vi "tb_fft test_host_sgl_2points.vi"() -> ()   [LabVIEW 2011]
uses:
  <userlib>/FPGA Library/Code Development/Signal Processing/FFT Block/FFT/Controls/FFT States.ctl
  <userlib>/FPGA Library/Code Development/Signal Processing/FFT Block/FFT/FFT Size.ctl
  <vilib>/Analysis/2dsp.llb/Real FFT.vi
  <vilib>/measure/maspectr.llb/FFT Spectrum (Mag-Phase) for 1 Chan (CDB).vi
  <vilib>/Analysis/1siggen.llb/Ramp Pattern by Samples.vi
  <vilib>/Analysis/NI_AALBase.lvlib
  <vilib>/measure/NI_MAPro.lvlib
  <vilib>/Analysis/NI_AALPro.lvlib
panel:
  out "xk_index":fxp<+,9,9>
  out "FFT Output Index":i32
  out "Current Index":u16
  out "Current State":T1=enum."Process"
  out "LabVIEW FPGA OUt":dbl[](array[numeric])
  out "LabVIEW":dbl[](array[numeric])
  out "Output":dbl[](array[numeric])
  out "Iterations Done":i32=550
  out "Pass?":bool=TRUE
  out "Error Signal":dbl[](graph)=[-2.3209475248815725e-14, 2.842170943040401e-14, -1.423246383868342e-14, -5.0290155712318274e-15, -5.617693635462835e-15, -1.2654220787659285e-14, -2.2653800450034258e-15, -7.817855587735912e-15, -5.642048551852787e-16, -4.848122315266641e-15, -1.4066308379314257e-15, -5.26182206995493e-15, -1.6787700245303399e-15, -3.5317597533564052e-15, -1.2179408859273234e-15, -5.682239243846926e-16, -1.476012201472354e-15, -4.387189911370367e-15, -4.712784380658982e-16, -1.1279118711067195e-15, -8.457455385367502e-16, -1.7591217350674133e-15, -1.2234105719754893e-15, -3.1796619632735843e-15, -1.1311752817825782e-15, -7.652138728201138e-16, -4.95475236507169e-16, -1.3804968391458857e-15, -6.200872213680143e-16, -1.6208905183375611e-15, -7.900785734892874e-16, -6.215416191232572e-15, -3.6014963741383564e-16, -6.5735506151035904e-15, -5.438526124809484e-16, -8.859964049951827e-16, -4.660820542011352e-16, -4.331250169872678e-16, -5.070423607357574e-16, -1.334222221931296e-15, -4.161038840225869e-16, -2.162642520615897e-15, -4.832602196126579e-16, -1.8466113911920694e-15, -5.111720910128212e-16, -1.3077661139157257e-15, -1.317295841380055e-16, -1.5344645445695557e-15, -5.003143032383381e-16, -8.907780307170318e-16, -3.4910614331552773e-16, -1.9659375815054982e-15, -2.522820868197333e-16, -1.3494997210405505e-15, -2.1367142635572254e-16, -1.2649677550390071e-15, -3.5078397942125153e-16, -1.493960591155926e-15, -3.7008746035102686e-16, -2.5695474807823932e-15, -2.1842124513731103e-16, -1.682876439042557e-15, -4.96013146890552e-16, -6.5726931140504286e-15, -2.3111578430367925e-16, -5.778724315304478e-15, -1.7672272640256473e-16, -2.3917285436809857e-15, -8.413654196767352e-17, -2.1045096122203425e-15, -2.324245509223888e-16, -2.1899677460894678e-15, -2.7245802781795665e-16, -1.0471757725153366e-15, -2.6086976997519237e-16, -2.7751674747999853e-15, -3.5068777984061774e-16, -1.4999120779771695e-15, -5.776639758822378e-17, -1.865769852058881e-15, -3.141749171548091e-16, -1.442932533559895e-15, -3.715679972475205e-16, -2.4873545340143905e-15, -3.0316037042699785e-16, -1.37060843732013e-15, -3.432134673273237e-17, -2.1823140172583753e-15, -3.2893911942517435e-16, -1.3802374497384821e-15, -2.515468723190618e-16, -2.0407080560795774e-15, -7.825246283752062e-17, -9.605012681453347e-16, -1.6665822022539347e-16, -8.585854605590916e-15, -8.279239838517457e-17, -8.029942062406046e-15, -2.549866803230553e-16, -1.3304883103107788e-15, -2.90011130209677e-16, -2.5843153744562437e-16, -3.0946190583309643e-16, -1.5925989429078613e-15, -1.9088697868535118e-16, -1.0709404142245489e-15, -1.863213961293967e-16, -1.401179966237845e-15, -4.025510697204942e-16, -3.065000004186774e-16, -2.4056748095016175e-16, -3.564162060583895e-15, -9.550773452918578e-17, -3.8814679519282134e-15, -6.671123007721539e-17, -5.082068342041713e-16, -1.8944012535004732e-16, -1.0775874498436763e-15, -2.0329123879890962e-16, -2.241124999344413e-15, -1.8315131472796022e-16, -2.5293144435025902e-15, -2.3090799989339955e-16, -2.612178765857882e-15, -7.52239796616572e-17, -1.3979455926566411e-15, -2.5913851848827294e-16, -7.112961996896967e-15, -2.225733614385263e-16, -7.158697954722229e-15, -2.1660085057067423e-16, -2.6486921612808084e-15, -6.056613111055876e-17, -2.288188675935301e-15, -2.574708219682569e-16, -9.746365606310544e-16, -2.5811420637914955e-16, -8.308310394594462e-16, -4.494030496521331e-17, -1.4914047073883096e-15, -1.2275946211757026e-16, -2.6789082049114747e-15, -7.646153710119143e-17, -3.614594974384435e-15, -1.5957370718388087e-16, -2.9071637037790352e-15, -1.0273012860538455e-16, -1.3529679760932233e-15, -2.1337438724207498e-16, -2.366087417632634e-15, -9.550540044778412e-17, -1.5267377900302278e-15, -1.0388147266081965e-16, -2.509352775164673e-15, -2.3294021415221696e-16, -1.5871319492314687e-15, -1.629641167659651e-16, -3.155068388354255e-15, -2.4295533381250624e-16, -1.789790942017654e-15, -2.1957682081227828e-16, -2.0620909489757014e-15, -2.636517897912316e-16, -3.19876498904266e-15, -4.76024074878868e-17, -2.8623217823864246e-15, -2.340225419378271e-16, -2.720367262450368e-15, -2.798717011154696e-16, -3.2704501244531444e-15, -8.294783416780197e-17, -4.3774499283332104e-15, -6.583259151313607e-17, -1.9123572024036315e-15, -8.859554359303103e-17, -3.909561650717318e-15, -2.157753926548324e-16, -2.631616832513605e-15, -1.8282424749852087e-16, -1.5012598370928595e-15, -2.6297488382582883e-16, -2.739819934401838e-16, -2.1835568909079528e-16, -4.566965697604556e-16, -2.844726135635231e-16, -6.029898128165984e-16, -4.031968136940985e-16, -1.2254274776086847e-15, -1.8567128477488958e-16, -1.2812099893063057e-15, -9.450275719635022e-17, -5.96208200198294e-15, -1.7413014862493185e-16, -6.362837003873818e-15, -3.8442560991005193e-16, -8.511897473684678e-16, -3.0298323627896944e-16, -6.374617717285576e-16, -3.980117316625464e-17, -1.889994438645939e-15, -7.924595323298657e-17, -1.1680802186811143e-15, -1.513694447821511e-16, -3.626366865071199e-16, -4.1911022380985105e-16, -1.5491215798532264e-15, -3.3152634782517783e-16, -1.0511118915755967e-15, -2.8375241753187317e-16, -3.0041210935611057e-15, -2.312884286263144e-16, -8.680462300544733e-16, -5.913378666039998e-16, -2.0124813913536014e-15, -4.849627295200987e-16, -3.0245786651048457e-15, -2.562926943075326e-16, -9.586214531000217e-16, -7.630416896386312e-17, -1.885296996390658e-15, -3.7641062798780547e-16, -1.3322161170514853e-15, -6.258042048959739e-16, -2.9484061140259706e-15, -2.478244140346566e-16, -4.381349750736086e-15, -3.055345357451583e-16, -8.254308413688034e-16, -2.1611396728793227e-16, -2.100174130362261e-15, -5.639679223541525e-16, -2.039042989477575e-15, -7.356320721078596e-16, -2.155129637976514e-15, -2.917622859196026e-16, -2.9817337018338868e-15, -5.901631083403165e-17, -1.4257302964464585e-15, -5.707161677436202e-16, -1.3123195162261534e-15, -1.3214037338257707e-15, -3.0060428009987197e-15, -9.650139214557572e-16, -2.010017297160963e-15, -9.477531974798123e-16, -4.598043857065251e-15, -1.2635405532302e-15, -5.575592142985788e-15, -1.2288406491237445e-15, -2.1260965321182736e-15, -1.1476659587055287e-15, -1.4004468922647886e-14, -1.8926642492776802e-15, -5.2356515256904374e-15, -7.733954207320486e-15, -3.0001115817680726e-14, -2.8911741707313143e-15, -3.0001115817680726e-14, -7.733954207320486e-15, -5.2356515256904374e-15, -1.8926642492776802e-15, -1.4004468922647886e-14, -1.1476659587055287e-15, -2.1260965321182736e-15, -1.2288406491237445e-15, -5.575592142985788e-15, -1.2635405532302e-15, -4.598043857065251e-15, -9.477531974798123e-16, -2.010017297160963e-15, -9.650139214557572e-16, -3.0060428009987197e-15, -1.3214037338257707e-15, -1.3123195162261534e-15, -5.707161677436202e-16, -1.4257302964464585e-15, -5.901631083403165e-17, -2.9817337018338868e-15, -2.917622859196026e-16, -2.155129637976514e-15, -7.356320721078596e-16, -2.039042989477575e-15, -5.639679223541525e-16, -2.100174130362261e-15, -2.1611396728793227e-16, -8.254308413688034e-16, -3.055345357451583e-16, -4.381349750736086e-15, -2.478244140346566e-16, -2.9484061140259706e-15, -6.258042048959739e-16, -1.3322161170514853e-15, -3.7641062798780547e-16, -1.885296996390658e-15, -7.630416896386312e-17, -9.586214531000217e-16, -2.562926943075326e-16, -3.0245786651048457e-15, -4.849627295200987e-16, -2.0124813913536014e-15, -5.913378666039998e-16, -8.680462300544733e-16, -2.312884286263144e-16, -3.0041210935611057e-15, -2.8375241753187317e-16, -1.0511118915755967e-15, -3.3152634782517783e-16, -1.5491215798532264e-15, -4.1911022380985105e-16, -3.626366865071199e-16, -1.513694447821511e-16, -1.1680802186811143e-15, -7.924595323298657e-17, -1.889994438645939e-15, -3.980117316625464e-17, -6.374617717285576e-16, -3.0298323627896944e-16, -8.511897473684678e-16, -3.8442560991005193e-16, -6.362837003873818e-15, -1.7413014862493185e-16, -5.96208200198294e-15, -9.450275719635022e-17, -1.2812099893063057e-15, -1.8567128477488958e-16, -1.2254274776086847e-15, -4.031968136940985e-16, -6.029898128165984e-16, -2.844726135635231e-16, -4.566965697604556e-16, -2.1835568909079528e-16, -2.739819934401838e-16, -2.6297488382582883e-16, -1.5012598370928595e-15, -1.8282424749852087e-16, -2.631616832513605e-15, -2.157753926548324e-16, -3.909561650717318e-15, -8.859554359303103e-17, -1.9123572024036315e-15, -6.583259151313607e-17, -4.3774499283332104e-15, -8.294783416780197e-17, -3.2704501244531444e-15, -2.798717011154696e-16, -2.720367262450368e-15, -2.340225419378271e-16, -2.8623217823864246e-15, -4.76024074878868e-17, -3.19876498904266e-15, -2.636517897912316e-16, -2.0620909489757014e-15, -2.1957682081227828e-16, -1.789790942017654e-15, -2.4295533381250624e-16, -3.155068388354255e-15, -1.629641167659651e-16, -1.5871319492314687e-15, -2.3294021415221696e-16, -2.509352775164673e-15, -1.0388147266081965e-16, -1.5267377900302278e-15, -9.550540044778412e-17, -2.366087417632634e-15, -2.1337438724207498e-16, -1.3529679760932233e-15, -1.0273012860538455e-16, -2.9071637037790352e-15, -1.5957370718388087e-16, -3.614594974384435e-15, -7.646153710119143e-17, -2.6789082049114747e-15, -1.2275946211757026e-16, -1.4914047073883096e-15, -4.494030496521331e-17, -8.308310394594462e-16, -2.5811420637914955e-16, -9.746365606310544e-16, -2.574708219682569e-16, -2.288188675935301e-15, -6.056613111055876e-17, -2.6486921612808084e-15, -2.1660085057067423e-16, -7.158697954722229e-15, -2.225733614385263e-16, -7.112961996896967e-15, -2.5913851848827294e-16, -1.3979455926566411e-15, -7.52239796616572e-17, -2.612178765857882e-15, -2.3090799989339955e-16, -2.5293144435025902e-15, -1.8315131472796022e-16, -2.241124999344413e-15, -2.0329123879890962e-16, -1.0775874498436763e-15, -1.8944012535004732e-16, -5.082068342041713e-16, -6.671123007721539e-17, -3.8814679519282134e-15, -9.550773452918578e-17, -3.564162060583895e-15, -2.4056748095016175e-16, -3.065000004186774e-16, -4.025510697204942e-16, -1.401179966237845e-15, -1.863213961293967e-16, -1.0709404142245489e-15, -1.9088697868535118e-16, -1.5925989429078613e-15, -3.0946190583309643e-16, -2.5843153744562437e-16, -2.90011130209677e-16, -1.3304883103107788e-15, -2.549866803230553e-16, -8.029942062406046e-15, -8.279239838517457e-17, -8.585854605590916e-15, -1.6665822022539347e-16, -9.605012681453347e-16, -7.825246283752062e-17, -2.0407080560795774e-15, -2.515468723190618e-16, -1.3802374497384821e-15, -3.2893911942517435e-16, -2.1823140172583753e-15, -3.432134673273237e-17, -1.37060843732013e-15, -3.0316037042699785e-16, -2.4873545340143905e-15, -3.715679972475205e-16, -1.442932533559895e-15, -3.141749171548091e-16, -1.865769852058881e-15, -5.776639758822378e-17, -1.4999120779771695e-15, -3.5068777984061774e-16, -2.7751674747999853e-15, -2.6086976997519237e-16, -1.0471757725153366e-15, -2.7245802781795665e-16, -2.1899677460894678e-15, -2.324245509223888e-16, -2.1045096122203425e-15, -8.413654196767352e-17, -2.3917285436809857e-15, -1.7672272640256473e-16, -5.778724315304478e-15, -2.3111578430367925e-16, -6.5726931140504286e-15, -4.96013146890552e-16, -1.682876439042557e-15, -2.1842124513731103e-16, -2.5695474807823932e-15, -3.7008746035102686e-16, -1.493960591155926e-15, -3.5078397942125153e-16, -1.2649677550390071e-15, -2.1367142635572254e-16, -1.3494997210405505e-15, -2.522820868197333e-16, -1.9659375815054982e-15, -3.4910614331552773e-16, -8.907780307170318e-16, -5.003143032383381e-16, -1.5344645445695557e-15, -1.317295841380055e-16, -1.3077661139157257e-15, -5.111720910128212e-16, -1.8466113911920694e-15, -4.832602196126579e-16, -2.162642520615897e-15, -4.161038840225869e-16, -1.334222221931296e-15, -5.070423607357574e-16, -4.331250169872678e-16, -4.660820542011352e-16, -8.859964049951827e-16, -5.438526124809484e-16, -6.5735506151035904e-15, -3.6014963741383564e-16, -6.215416191232572e-15, -7.900785734892874e-16, -1.6208905183375611e-15, -6.200872213680143e-16, -1.3804968391458857e-15, -4.95475236507169e-16, -7.652138728201138e-16, -1.1311752817825782e-15, -3.1796619632735843e-15, -1.2234105719754893e-15, -1.7591217350674133e-15, -8.457455385367502e-16, -1.1279118711067195e-15, -4.712784380658982e-16, -4.387189911370367e-15, -1.476012201472354e-15, -5.682239243846926e-16, -1.2179408859273234e-15, -3.5317597533564052e-15, -1.6787700245303399e-15, -5.26182206995493e-15, -1.4066308379314257e-15, -4.848122315266641e-15, -5.642048551852787e-16, -7.817855587735912e-15, -2.2653800450034258e-15, -1.2654220787659285e-14, -5.617693635462835e-15, -5.0290155712318274e-15, -1.423246383868342e-14, 2.842170943040401e-14]
  out "FFT_FLP_LabVIEW":dbl[](graph)
  out "LabVIEW FPGA":dbl[](graph)=[0.0, 256.0, 0.0, 0.0, 0.0, 0.0, 0.0, 0.0, 0.0, 0.0, 0.0, 0.0, 0.0, 0.0, 0.0, 0.0, 0.0, 0.0, 0.0, 0.0, 0.0, 0.0, 0.0, 0.0, 0.0, 0.0, 0.0, 0.0, 0.0, 0.0, 0.0, 0.0, 0.0, 0.0, 0.0, 0.0, 0.0, 0.0, 0.0, 0.0, 0.0, 0.0, 0.0, 0.0, 0.0, 0.0, 0.0, 0.0, 0.0, 0.0, 0.0, 0.0, 0.0, 0.0, 0.0, 0.0, 0.0, 0.0, 0.0, 0.0, 0.0, 0.0, 0.0, 0.0, 0.0, 0.0, 0.0, 0.0, 0.0, 0.0, 0.0, 0.0, 0.0, 0.0, 0.0, 0.0, 0.0, 0.0, 0.0, 0.0, 0.0, 0.0, 0.0, 0.0, 0.0, 0.0, 0.0, 0.0, 0.0, 0.0, 0.0, 0.0, 0.0, 0.0, 0.0, 0.0, 0.0, 0.0, 0.0, 0.0, 0.0, 0.0, 0.0, 0.0, 0.0, 0.0, 0.0, 0.0, 0.0, 0.0, 0.0, 0.0, 0.0, 0.0, 0.0, 0.0, 0.0, 0.0, 0.0, 0.0, 0.0, 0.0, 0.0, 0.0, 0.0, 0.0, 0.0, 0.0, 0.0, 0.0, 0.0, 0.0, 0.0, 0.0, 0.0, 0.0, 0.0, 0.0, 0.0, 0.0, 0.0, 0.0, 0.0, 0.0, 0.0, 0.0, 0.0, 0.0, 0.0, 0.0, 0.0, 0.0, 0.0, 0.0, 0.0, 0.0, 0.0, 0.0, 0.0, 0.0, 0.0, 0.0, 0.0, 0.0, 0.0, 0.0, 0.0, 0.0, 0.0, 0.0, 0.0, 0.0, 0.0, 0.0, 0.0, 0.0, 0.0, 0.0, 0.0, 0.0, 0.0, 0.0, 0.0, 0.0, 0.0, 0.0, 0.0, 0.0, 0.0, 0.0, 0.0, 0.0, 0.0, 0.0, 0.0, 0.0, 0.0, 0.0, 0.0, 0.0, 0.0, 0.0, 0.0, 0.0, 0.0, 0.0, 0.0, 0.0, 0.0, 0.0, 0.0, 0.0, 0.0, 0.0, 0.0, 0.0, 0.0, 0.0, 0.0, 0.0, 0.0, 0.0, 0.0, 0.0, 0.0, 0.0, 0.0, 0.0, 0.0, 0.0, 0.0, 0.0, 0.0, 0.0, 0.0, 0.0, 0.0, 0.0, 0.0, 0.0, 0.0, 0.0, 0.0, 0.0, 0.0, 0.0, 0.0, 0.0, 0.0, 0.0, 0.0, 0.0, 0.0, 0.0, 0.0, 0.0, 0.0, 0.0, 0.0, 0.0, 0.0, 0.0, 0.0, 0.0, 0.0, 0.0, 0.0, 0.0, 0.0, 0.0, 0.0, 0.0, 0.0, 0.0, 0.0, 0.0, 0.0, 0.0, 0.0, 0.0, 0.0, 0.0, 0.0, 0.0, 0.0, 0.0, 0.0, 0.0, 0.0, 0.0, 0.0, 0.0, 0.0, 0.0, 0.0, 0.0, 0.0, 0.0, 0.0, 0.0, 0.0, 0.0, 0.0, 0.0, 0.0, 0.0, 0.0, 0.0, 0.0, 0.0, 0.0, 0.0, 0.0, 0.0, 0.0, 0.0, 0.0, 0.0, 0.0, 0.0, 0.0, 0.0, 0.0, 0.0, 0.0, 0.0, 0.0, 0.0, 0.0, 0.0, 0.0, 0.0, 0.0, 0.0, 0.0, 0.0, 0.0, 0.0, 0.0, 0.0, 0.0, 0.0, 0.0, 0.0, 0.0, 0.0, 0.0, 0.0, 0.0, 0.0, 0.0, 0.0, 0.0, 0.0, 0.0, 0.0, 0.0, 0.0, 0.0, 0.0, 0.0, 0.0, 0.0, 0.0, 0.0, 0.0, 0.0, 0.0, 0.0, 0.0, 0.0, 0.0, 0.0, 0.0, 0.0, 0.0, 0.0, 0.0, 0.0, 0.0, 0.0, 0.0, 0.0, 0.0, 0.0, 0.0, 0.0, 0.0, 0.0, 0.0, 0.0, 0.0, 0.0, 0.0, 0.0, 0.0, 0.0, 0.0, 0.0, 0.0, 0.0, 0.0, 0.0, 0.0, 0.0, 0.0, 0.0, 0.0, 0.0, 0.0, 0.0, 0.0, 0.0, 0.0, 0.0, 0.0, 0.0, 0.0, 0.0, 0.0, 0.0, 0.0, 0.0, 0.0, 0.0, 0.0, 0.0, 0.0, 0.0, 0.0, 0.0, 0.0, 0.0, 0.0, 0.0, 0.0, 0.0, 0.0, 0.0, 0.0, 0.0, 0.0, 0.0, 0.0, 0.0, 0.0, 0.0, 0.0, 0.0, 0.0, 0.0, 0.0, 0.0, 0.0, 0.0, 0.0, 0.0, 0.0, 0.0, 0.0, 0.0, 0.0, 0.0, 0.0, 0.0, 0.0, 0.0, 0.0, 0.0, 0.0, 0.0, 0.0, 0.0, 0.0, 0.0, 0.0, 0.0, 0.0, 0.0, 0.0, 0.0, 0.0, 0.0, 0.0, 0.0, 0.0, 0.0, 0.0, 0.0, 0.0, 0.0, 0.0, 0.0, 0.0, 0.0, 0.0, 0.0, 0.0, 0.0, 0.0, 0.0, 0.0, 0.0, 0.0, 0.0, 0.0, 0.0, 0.0, 0.0, 0.0, 0.0, 256.0]
  out "Error Spectrum":cluster{"f0":dbl, "df":dbl, "magnitude":dbl[]}(graph)={"f0"=-0.5, "df"=0.001953125, "magnitude"=[-298.08911652616155, -303.0581849455438, -315.41253856942467, -312.4872641856872, -310.42255535927274, -310.26035064488815, -310.73498931783695, -311.58984667376325, -311.9691048373197, -313.22613406670905, -314.05897490696896, -312.6090821162051, -311.38107609426964, -312.4480515707975, -316.4975935715534, -313.28623370551855, -309.3480811605718, -311.8765354467341, -313.7191966512445, -313.44164506805885, -319.67876893815014, -326.2042803276112, -318.3336994066264, -313.20507803727867, -311.7500738342471, -313.7293886931966, -321.0385961638018, -330.9036814978236, -323.8666157001631, -321.8743668527293, -327.81900883460816, -315.56431828444465, -310.56326288194265, -317.99456951046545, -342.8853731100542, -322.3070045592143, -321.58376270277483, -327.87595550984656, -323.85601241806086, -318.51067005273853, -317.4232218058295, -318.66603209592677, -325.8698473189381, -339.6450070239324, -322.95282360998317, -316.46091509942556, -319.0283626780748, -318.11551777988035, -313.5225877610049, -316.38435900508534, -320.15487376867713, -320.72689062496687, -324.62121035524774, -323.30243906554443, -320.1440042571933, -321.0819800286996, -321.5348875995385, -320.46015197418785, -335.0938698298407, -328.02619077036593, -331.6753516058508, -323.4770128228402, -330.1403040872466, -318.7545112106158, -312.484631392163, -317.33658959636875, -327.43407086896207, -321.892199597669, -326.0109585414713, -334.02781625259195, -330.3647312798665, -317.0463451787754, -315.97386536191283, -318.2450107053468, -322.0601825458229, -326.3539921027293, -323.1549948609168, -318.6053369700705, -319.16797092381813, -318.29055884458194, -315.8830692860334, -318.54158341817106, -318.8417128260067, -316.9223858814386, -319.58968853761553, -321.87968487322854, -320.7039418824355, -317.9492392378816, -315.42522063331256, -315.24596872730444, -317.4427233805529, -320.52308232479623, -319.15876262337764, -317.4746786167459, -317.77852033266447, -313.7782996973245, -310.51739194105124, -312.0511191533593, -313.39377896336833, -311.8081564540838, -312.2109755866337, -314.5335662631336, -315.5893804499518, -314.8343793462807, -315.49973993812443, -317.2062266395026, -317.99121732253235, -316.62309071189776, -315.1147370965974, -314.50836215554494, -315.20750626153824, -315.41187486316267, -314.72307267564696, -315.56175868412225, -315.8609532502685, -316.7277503556269, -320.4969625327314, -323.214983580055, -320.6033311461665, -317.78969449101953, -317.19952632625285, -319.2419145530334, -325.30662185326497, -329.69255177156765, -323.9120348364795, -326.1396196955613, -331.73888138492464, -325.1950453333449, -328.6841566766478, -334.2723425189815, -326.2760021682447, -331.2424420475836, -335.44717993622874, -326.4943280721517, -332.7821158187069, -329.8585992854489, -323.77874523933775, -324.2840113485023, -333.0055265694674, -344.9935006708449, -333.87605704018284, -323.06447522272805, -321.42237642800575, -322.0443271626987, -321.44363604784144, -321.11640243002427, -319.79113947555, -318.77882825371256, -319.66957511800626, -322.2687593824885, -324.6257012061602, -322.6378858832113, -319.2767399904177, -318.14331817298853, -319.26378136880373, -317.6490079846138, -314.62493301930925, -314.1835138827547, -316.24384226273486, -314.42819430688115, -312.50861713568577, -316.6571200773707, -322.43794033493003, -321.78889533998614, -324.18269104660897, -326.52486135211313, -321.19335663781163, -317.7892377961542, -317.8636218113048, -321.4748614760423, -325.8048641302873, -328.29883895954265, -324.70019470195075, -320.4379006177755, -323.216876849234, -322.5968447372005, -318.5189210320941, -323.23572671288184, -326.8471902012731, -322.9172220005846, -329.0534987442593, -337.11049564944636, -326.1527024150165, -320.27035622614676, -317.19213339135075, -318.14774937454007, -334.4427785848869, -331.0805596952952, -326.5749628598911, -321.7992991932838, -326.53145324446, -316.53059030585484, -311.7711008255268, -317.1515761486268, -324.46226333810773, -319.8287768467248, -322.3735599579331, -332.51422237443, -323.69161166867855, -318.17771976470686, -319.90966795720533, -321.333789165993, -321.86880297709047, -323.72577405855657, -322.8812209888758, -319.10180211793715, -318.1401659695759, -314.7533487212259, -312.0948197662708, -315.54257809162056, -316.0038825426357, -313.90921041047994, -317.9838157912971, -322.499767911265, -317.78896532767635, -314.21192478861514, -313.54783263954937, -314.2498866005032, -317.0737045560749, -318.3366878301345, -315.50895772132446, -315.583461680881, -319.6144843867234, -313.10223960456335, -308.290144923361, -311.94429231109547, -318.16382305331877, -315.807239419594, -316.7621912952867, -319.0400011622606, -315.40678032148287, -310.9301676756224, -309.1827648396873, -310.06903486973897, -313.2118410749616, -316.20049270843117, -313.73950076092603, -310.4977273177817, -310.686632833173, -308.9764172824766, -306.8408831548783, -309.3431909742103, -311.01114793861086, -308.45303726486515, -307.58895732291654, -308.15097238160905, -308.87389874981176, -308.25946568069617, -307.35499070320327, -306.84127804500883, -306.2221447850663, -305.7270122705749, -305.51080676376154, -306.0015281763568, -306.78919624998105, -299.2564245504833, -295.1671121878411, -299.2564245504833, -306.78919624998105, -306.0015281763568, -305.51080676376154, -305.7270122705749, -306.2221447850663, -306.84127804500883, -307.35499070320327, -308.25946568069617, -308.87389874981176, -308.15097238160905, -307.58895732291654, -308.45303726486515, -311.01114793861086, -309.3431909742103, -306.8408831548783, -308.9764172824766, -310.68663283317306, -310.4977273177817, -313.73950076092603, -316.20049270843117, -313.2118410749616, -310.06903486973897, -309.1827648396873, -310.9301676756224, -315.4067803214829, -319.0400011622606, -316.7621912952867, -315.807239419594, -318.16382305331877, -311.94429231109547, -308.290144923361, -313.10223960456335, -319.6144843867234, -315.583461680881, -315.50895772132446, -318.33668783013457, -317.0737045560749, -314.2498866005032, -313.54783263954937, -314.21192478861514, -317.78896532767635, -322.499767911265, -317.9838157912971, -313.90921041047994, -316.0038825426357, -315.54257809162056, -312.0948197662708, -314.7533487212259, -318.1401659695759, -319.10180211793715, -322.8812209888758, -323.72577405855657, -321.86880297709047, -321.333789165993, -319.9096679572054, -318.17771976470686, -323.69161166867855, -332.51422237443, -322.3735599579331, -319.8287768467248, -324.46226333810773, -317.1515761486268, -311.7711008255268, -316.53059030585484, -326.53145324446, -321.7992991932838, -326.57496285989106, -331.0805596952952, -334.4427785848869, -318.14774937454, -317.19213339135075, -320.27035622614676, -326.1527024150165, -337.11049564944636, -329.0534987442593, -322.9172220005846, -326.8471902012731, -323.2357267128819, -318.5189210320941, -322.5968447372005, -323.216876849234, -320.4379006177755, -324.70019470195075, -328.29883895954265, -325.8048641302873, -321.4748614760423, -317.8636218113048, -317.7892377961542, -321.19335663781163, -326.524861352113, -324.18269104660897, -321.78889533998614, -322.43794033493003, -316.6571200773707, -312.50861713568577, -314.42819430688115, -316.24384226273486, -314.1835138827547, -314.62493301930925, -317.6490079846138, -319.26378136880373, -318.14331817298853, -319.2767399904177, -322.6378858832113, -324.6257012061602, -322.2687593824885, -319.66957511800626, -318.77882825371256, -319.79113947555, -321.11640243002427, -321.44363604784144, -322.0443271626987, -321.42237642800575, -323.06447522272805, -333.87605704018284, -344.99350067084487, -333.0055265694674, -324.2840113485024, -323.77874523933775, -329.8585992854489, -332.7821158187069, -326.4943280721517, -335.44717993622874, -331.24244204758355, -326.2760021682447, -334.2723425189815, -328.6841566766478, -325.1950453333449, -331.73888138492464, -326.1396196955613, -323.9120348364795, -329.69255177156765, -325.30662185326497, -319.2419145530334, -317.19952632625285, -317.78969449101953, -320.6033311461665, -323.214983580055, -320.4969625327314, -316.7277503556269, -315.8609532502685, -315.56175868412225, -314.72307267564696, -315.41187486316267, -315.20750626153824, -314.50836215554494, -315.1147370965974, -316.62309071189776, -317.9912173225323, -317.2062266395026, -315.49973993812443, -314.8343793462807, -315.5893804499518, -314.5335662631336, -312.2109755866337, -311.8081564540838, -313.39377896336833, -312.0511191533593, -310.51739194105124, -313.7782996973245, -317.77852033266447, -317.4746786167459, -319.15876262337764, -320.52308232479623, -317.4427233805529, -315.24596872730444, -315.42522063331256, -317.9492392378816, -320.7039418824355, -321.87968487322854, -319.58968853761553, -316.9223858814386, -318.8417128260067, -318.54158341817106, -315.8830692860334, -318.29055884458194, -319.16797092381813, -318.6053369700705, -323.1549948609168, -326.3539921027293, -322.0601825458229, -318.2450107053468, -315.97386536191283, -317.0463451787754, -330.3647312798665, -334.02781625259195, -326.0109585414713, -321.892199597669, -327.43407086896207, -317.33658959636875, -312.484631392163, -318.7545112106158, -330.1403040872466, -323.47701282284015, -331.6753516058508, -328.02619077036604, -335.0938698298407, -320.46015197418774, -321.5348875995385, -321.0819800286996, -320.1440042571933, -323.30243906554443, -324.62121035524774, -320.72689062496687, -320.15487376867713, -316.38435900508534, -313.5225877610049, -318.11551777988035, -319.0283626780748, -316.46091509942556, -322.95282360998317, -339.6450070239324, -325.8698473189381, -318.66603209592677, -317.4232218058295, -318.51067005273853, -323.85601241806086, -327.87595550984656, -321.58376270277483, -322.3070045592143, -342.8853731100542, -317.99456951046545, -310.56326288194265, -315.5643182844446, -327.8190088346081, -321.8743668527293, -323.8666157001631, -330.9036814978235, -321.0385961638018, -313.72938869319654, -311.7500738342471, -313.20507803727867, -318.3336994066264, -326.2042803276112, -319.67876893815014, -313.44164506805885, -313.7191966512445, -311.8765354467341, -309.3480811605718, -313.28623370551855, -316.4975935715534, -312.4480515707975, -311.38107609426964, -312.6090821162051, -314.05897490696896, -313.22613406670905, -311.9691048373197, -311.58984667376325, -310.73498931783695, -310.26035064488815, -310.42255535927274, -312.4872641856872, -315.41253856942467, -303.0581849455438]}
  in  "Stimulus Type":enum16{"Sine", "Ramp", "Chirp"}(ring)
  in  "Samples":u16=2048
  out "RMS Error":dbl=9.646094565272268e-13
  out "Max Error (dB)":dbl=295.1671121878411
  # "Stimulus"
  # "Error"
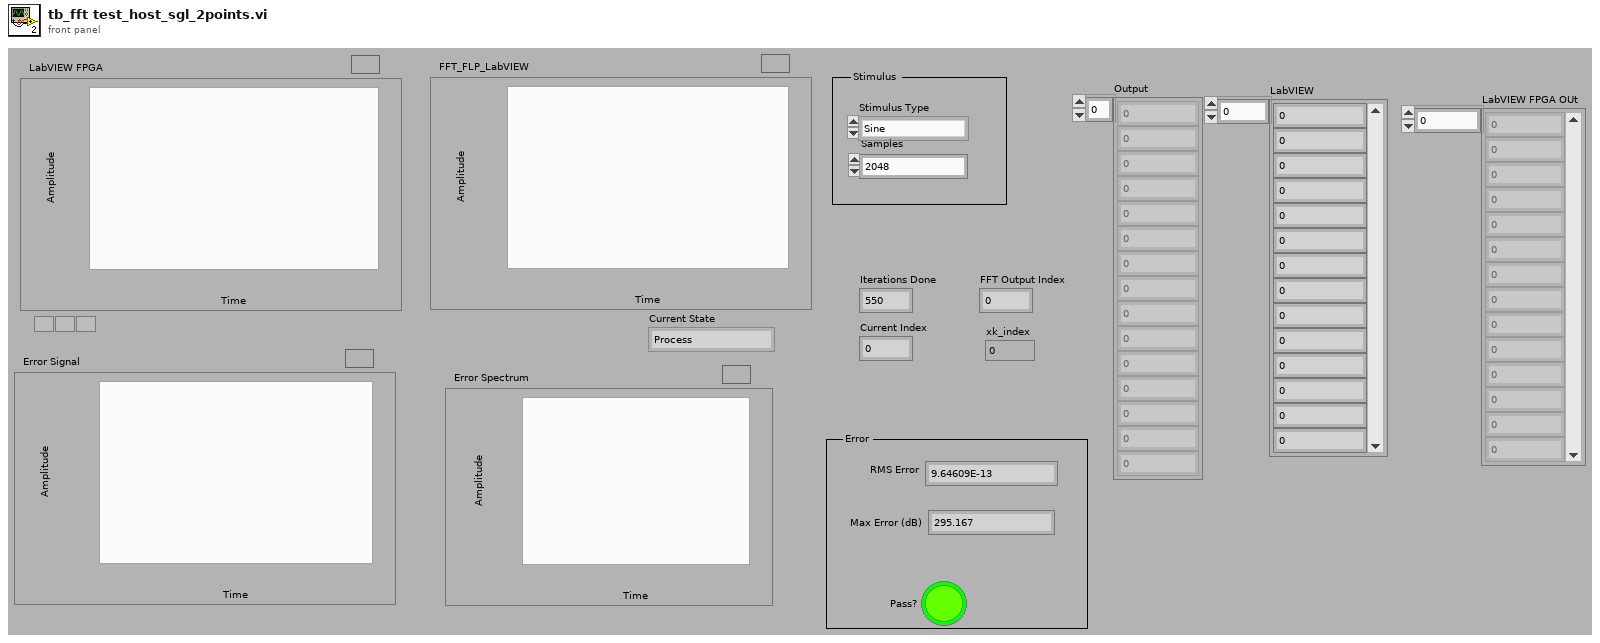
[diagram p1: front panel]
types:
  T1 = typedef "FFT States.ctl" = enum8{"Configure", "Start FFT processing", "Process", "Unload Last FFT", "Reset"}
  T2 = cluster{"dB On (F)":bool, "unwrap phase (F)":bool, "convert to degree (F)":bool}
  T3 = typedef "FFT Size.ctl" = enum16{"32", "64", "128", "256", "512", "1024", "2048", "4096", "8192", "16384", "32768", "65536"}
  T4 = cluster{"Reset":bool, "Start FFT":bool, "fwd_inv_we":bool, "fwd_inv":bool}
  T5 = cluster{"xk_im":fxp<+,32,32>, "xk_re":fxp<+,32,32>}
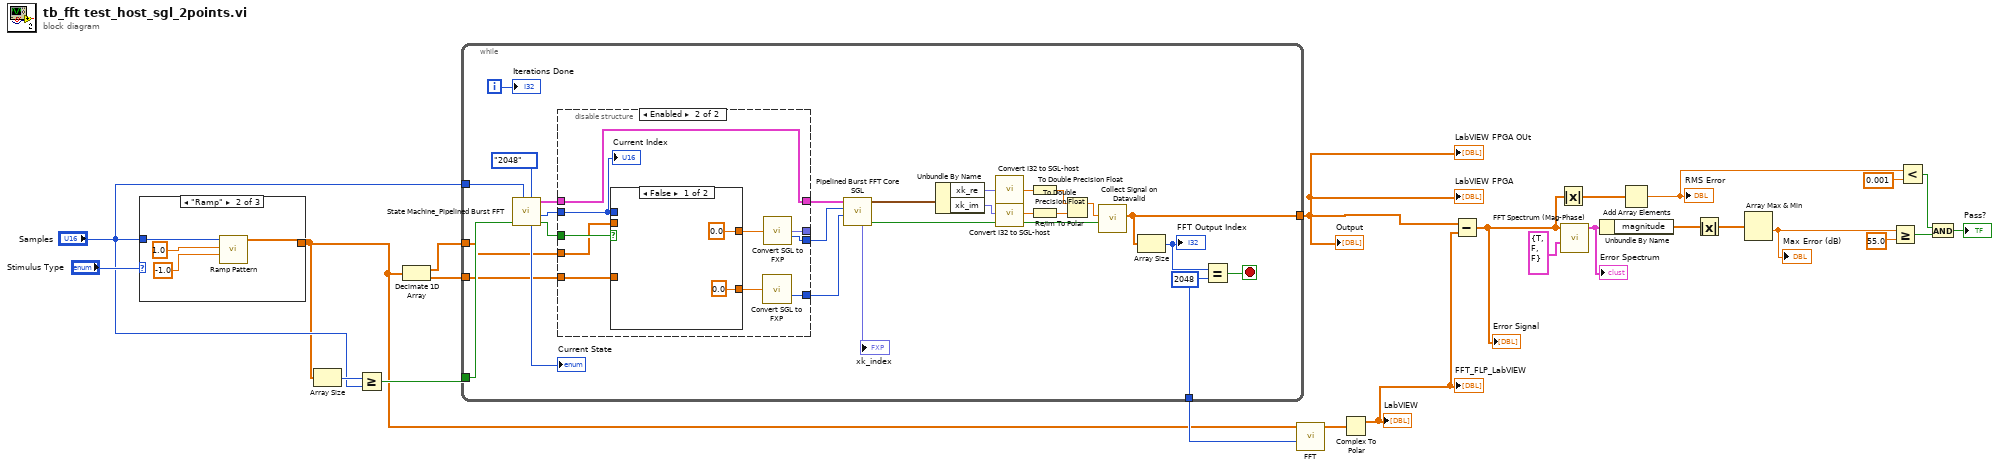
[diagram p0: block diagram]
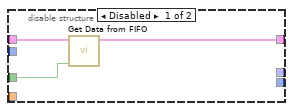
[diagram p2: hidden frame]
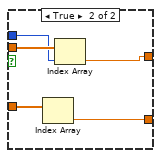
[diagram p3: hidden frame]
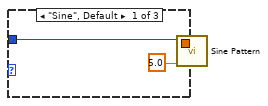
[diagram p4: hidden frame]
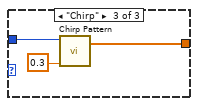
[diagram p5: hidden frame]
diagram:
  n1 = case shown="\"Ramp\"" "Stimulus Type" {
    tunnel: "Samples" -> [w27 w29 w34]
    tunnel: [w25 w28 w32] -> w3
    frame "Sine", Default {
      n2 = call <vilib>:"Sine Pattern.vi"("cycles"=5.0, "samples"=w27) -> ("Sinusoidal Pattern"=w25:dbl[])  [unwired: 2 in, 1 out]
    }
    frame "Ramp" {
      n3 = call-poly <vilib>:"Ramp Pattern.vi"("start"=-1.0, "end"=1.0, "samples"=w29) -> ("Ramp Pattern"=w28:dbl[])  [unwired: 7 in, 1 out]
    }
    frame "Chirp" {
      n4 = call <vilib>:"Chirp Pattern.vi"("f2"=0.3, "samples"=w34) -> ("Chirp Pattern"=w32:dbl[])  [unwired: 2 in, 1 out]
    }
  }
  n5 = Array Size(array=w3) -> (size(s)=w7:i32)
  n6 = Greater Or Equal?(x=w7, y="Samples") -> (x >= y?=w6:bool)
  n7 = Decimate 1D Array(w3) -> (w2:dbl[], w1:dbl[])
  n8 = while {
    tunnel: [w58] -> w17
    tunnel: w6 -> [w51]
    tunnel: "Samples" -> [w52]
    tunnel: w2 -> [w47]
    tunnel: [w41] -> w4
    tunnel: w1 -> [w36]
    i -> [w59]
    stop <- w57 stop-if-true
    w41 = 2048 ("y")
    n9 = call <userlib>:"State Machine_Pipelined Burst FFT.vi"("FFT Size"=FFT_Size."2048", "Required FFT Length"=w52, "Start FFT (New Record)"=w51) -> ("Get New Data"=w48:bool, "Current Index"=w46:u16, "State Info"=w49:T4, "FFT SM Current State"=→"Current State":T1)  [unwired: 5 in]
    n10 = disable-structure shown="Enabled" {
      disable-tunnel: w49 -> [w64 w73]
      disable-tunnel: w48 -> [w63 w74]
      disable-tunnel: [w62 w73] -> w45
      disable-tunnel: w47 -> [_ w72]
      disable-tunnel: [_ w70] -> _
      disable-tunnel: w46 -> [_ w69]
      disable-tunnel: [_ w68] -> w40
      disable-tunnel: w36 -> [_ w67]
      disable-tunnel: [_ w65] -> w35
      frame Disabled {
        n11 = call <userlib>:"Get Data from FIFO.vi"("Get New Data"=w63, "FFT State Info"=w64) -> ("FFT State Info Out"=w62:T4)  [unwired: 7 in, 2 out]
      }
      frame Enabled {
        n12 = case shown="False" w74 {
          tunnel: [0.0 w81] -> w71
          tunnel: w72 -> [_ w80]
          tunnel: w69 -> [_ w79]
          tunnel: w67 -> [_ w78]
          tunnel: [0.0 w77] -> w66
          frame False {
          }
          frame True {
            n13 = Index Array(array=w78) -> (element=w77:dbl)  [unwired: 1 in]
            n14 = Index Array(array=w80, index=w79) -> (element=w81:dbl)
          }
        }
        n15 = call <userlib>:"Convert SGL to FXP.vi"("Input"=w66) -> ("I32"=w65:i32)  [unwired: 12 in, 2 out]
        n16 = call <userlib>:"Convert SGL to FXP.vi"("Input"=w71) -> ("FXP Output"=w70:fxp<+,32,32>, "I32"=w68:i32)  [unwired: 12 in, 1 out]
        "Current Index" <- w69
      }
    }
    n17 = call <userlib>:"Pipelined Burst FFT Core SGL.vi"("xn_im"=w35, "xn_re"=w40, "FFT State Info In"=w45) -> ("Output Valid"=w44:bool, "FFT Output"=w39:T5, "xk_index"=→"xk_index":fxp<+,9,9>)  [unwired: 3 in, 3 out]
    n18 = Unbundle By Name(w39) -> ("xk_re"=w38:fxp<+,32,32>, "xk_im"=w37:fxp<+,32,32>)
    n19 = call <userlib>:"Convert I32 to SGL-host.vi"("Input"=w38) -> ("Output SGL"=w60:sgl)  [unwired: 14 in]
    n20 = call <userlib>:"Convert I32 to SGL-host.vi"("Input"=w37) -> ("Output SGL"=w61:sgl)  [unwired: 14 in]
    n21 = To Double Precision Float(number=w60) -> (double precision float=w54:dbl)
    n22 = To Double Precision Float(number=w61) -> (double precision float=w53:dbl)
    n23 = Re/Im To Polar(2:w53, 3:w54) -> (1:w55:dbl)  [unwired: 1 out]
    n24 = call <userlib>:"Collect Signal on Datavalid.vi"("Data Valid"=w44, "Input"=w55) -> ("Output"=w58:dbl[])  [unwired: 9 in]
    n25 = Array Size(array=w58) -> (size(s)=w56:i32)
    "FFT Output Index" <- w56
    n26 = Equal?(x=w56, y=w41) -> (x = y?=w57:bool)
    "Iterations Done" <- w59
  }
  "LabVIEW FPGA" <- w17
  "Output" <- w17
  "LabVIEW FPGA OUt" <- w17
  n27 = call-poly <vilib>:"FFT.vi"("FFT size"=w4, "X"=w3) -> ("FFT {X}"=w20:cdb[])  [unwired: 8 in, 1 out]
  n28 = Complex To Polar(r * e^(i*theta)=w20) -> (r=w16:dbl[])  [unwired: 1 out]
  "FFT_FLP_LabVIEW" <- w16
  "LabVIEW" <- w16
  n29 = Subtract(x=w17, y=w16) -> (x-y=w15:dbl[])
  "Error Signal" <- w15
  n30 = Absolute Value(x=w15) -> (abs(x)=w21:dbl[])
  n31 = call-poly <vilib>:"FFT Spectrum (Mag-Phase).vi"("view"=T2 {"dB On (F)"=TRUE, "unwrap phase (F)"=FALSE, "convert to degree (F)"=FALSE}, "time signal"=w15) -> ("magnitude"=w18:cluster{"f0":dbl, "df":dbl, "magnitude":dbl[]})  [unwired: 5 in, 4 out]
  "Error Spectrum" <- w18
  n32 = Unbundle By Name(w18) -> ("magnitude"=w23:dbl[])
  n33 = Add Array Elements(numeric array=w21) -> (sum=w12:dbl)
  "RMS Error" <- w12
  n34 = Absolute Value(x=w23) -> (abs(x)=w22:dbl[])
  n35 = Array Max & Min(array=w22) -> (min value=w14:dbl)  [unwired: 3 out]
  "Max Error (dB)" <- w14
  n36 = Greater Or Equal?(x=w14, y=55.0) -> (x >= y?=w9:bool)
  n37 = Less?(x=w12, y=0.001) -> (x < y?=w10:bool)
  n38 = And(x=w10, y=w9) -> (x .and. y?=→"Pass?":bool)
